vi "Read_Config.vi"(0 "GPIO 1 Config":enum32{"Off", "Read", "Write", "PWM "}(radio), 1 "GPIO 2 Config":enum32{"Off", "Read", "Write", "PWM "}(radio), 2 "GPIO 3 Config":enum32{"Off", "Read", "Write", "PWM "}(radio), 3 "Battery_Config":u16(ring)=1 items=["Off", "On"], 6 "Analog 1 Config":enum32{"Analog Read", "Off"}(radio), 10 "Analog 2 Config":enum32{"Analog Read", "Off"}(radio), 11 "Analog 3 Config":enum32{"Analog Read", "Off"}(radio), 14 "Error In":errorcluster, 15 "LINX Resource":T1) -> (18 "Read_Config":i32[](array[numeric]), 19 "Voltage":dbl(slide) caption="Tank" scale=3.0..6.0, 20 "GPIO 1 Read":bool, 21 "Analog 2":dbl, 22 "GPIO 2 Read":bool, 23 "Analog 3":dbl, 24 "GPIO 3 Read":bool, 25 "Error Out":errorcluster, 26 "Analog 1":dbl, 27 "LINX Resource 2":T1)   [LabVIEW 2018, in "ArgoBotLib.lvlib"]
uses:
  ArgoBotLib.lvlib
  <vilib>/MakerHub/LINX/Private/Type Defs/LINX Ref.ctl
  <vilib>/MakerHub/LINX/Private/Type Defs/Platform.ctl
  <vilib>/MakerHub/LINX/Private/Type Defs/Interface.ctl
  <vilib>/MakerHub/LINX/Private/Device/Type Defs/LINX Device Config.ctl
  <vilib>/MakerHub/LINX/Private/Device/Type Defs/TCP Config.ctl
  <vilib>/MakerHub/LINX/Private/Device/Type Defs/Channels.ctl
  <vilib>/MakerHub/LINX/Public/Peripherals/Digital/Digital Read N Chans.vi
  <vilib>/MakerHub/LINX/Public/Peripherals/Analog/Analog Read N Chans.vi
  <vilib>/MakerHub/LINX/Private/Local IO/LinxDigitalRead.vi
  <vilib>/MakerHub/LINX/Public/Utilities/Check Channel.vi
  <vilib>/MakerHub/LINX/Private/Local IO/LinxAnalogRead.vi
  <vilib>/MakerHub/LINX/Private/Utilties/Generate Error.vi
  <vilib>/MakerHub/LINX/LMH-LINX.lvlib
  <vilib>/MakerHub/LINX/Private/Device/Device.lvlib
panel:
  # "ArgoBot Read Config"
  # "This vi configures and reads the gpio and analog channels"
  # "Inputs"
  # "Outputs"
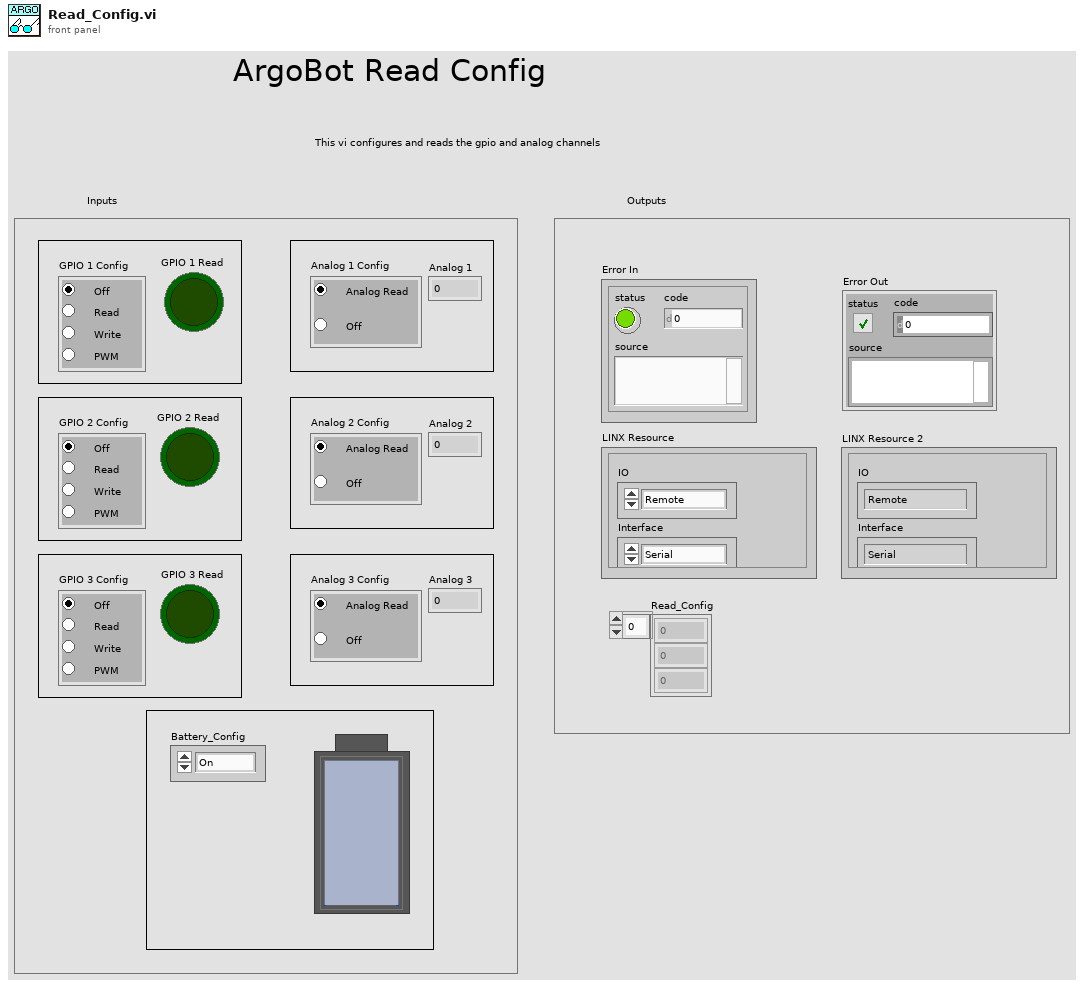
[diagram p1: front panel]
types:
  T1 = typedef "LMH-LINX.lvlib/LINX Ref.ctl" = cluster{"IO":T2, "Interface":T3, "LINX Device Config":T4}
  T2 = typedef "LMH-LINX.lvlib/Platform.ctl" = enum16{"Remote", "Local"}
  T3 = typedef "LMH-LINX.lvlib/Interface.ctl" = enum16{"Serial", "TCP"}
  T4 = typedef "LMH-LINX.lvlib/Device.lvlib/LINX Device Config.ctl" = cluster{"Interface":T3, "COM Port":refnum<visa-resource-name>, "TCP Configuration":T5, "Device Family":u8, "Device ID":u8, "Device Name":string, "TCP Ref":refnum<k5>, "Channels":T6}
  T5 = typedef "LMH-LINX.lvlib/Device.lvlib/TCP Config.ctl" = cluster{"IP Address":string, "Port":u16}
  T6 = typedef "LMH-LINX.lvlib/Channels.ctl" = cluster{"DI":u8[], "DO":u8[], "AI":u8[], "AO":u8[], "PWM":u8[], "QE":u8[], "UART":u8[], "I2C 2":u8[], "SPI":u8[], "CAN":u8[], "Servo":u8[], "AI Ref (V)":dbl, "AI Resolution (Bits)":u8, "AO Ref (V)":dbl, "AO Resolution (Bits)":u8}
  T7 = cluster{"GPIO 1 Config":enum32{"Off", "Read", "Write", "PWM "}, "GPIO 2 Config":enum32{"Off", "Read", "Write", "PWM "}, "GPIO 3 Config":enum32{"Off", "Read", "Write", "PWM "}, "Analog 1 Config":enum32{"Analog Read", "Off"}, "Analog 2 Config":enum32{"Analog Read", "Off"}, "Analog 3 Config":enum32{"Analog Read", "Off"}, "Battery_Config":u16, "LINX Resource":T1, "Error In":errorcluster}
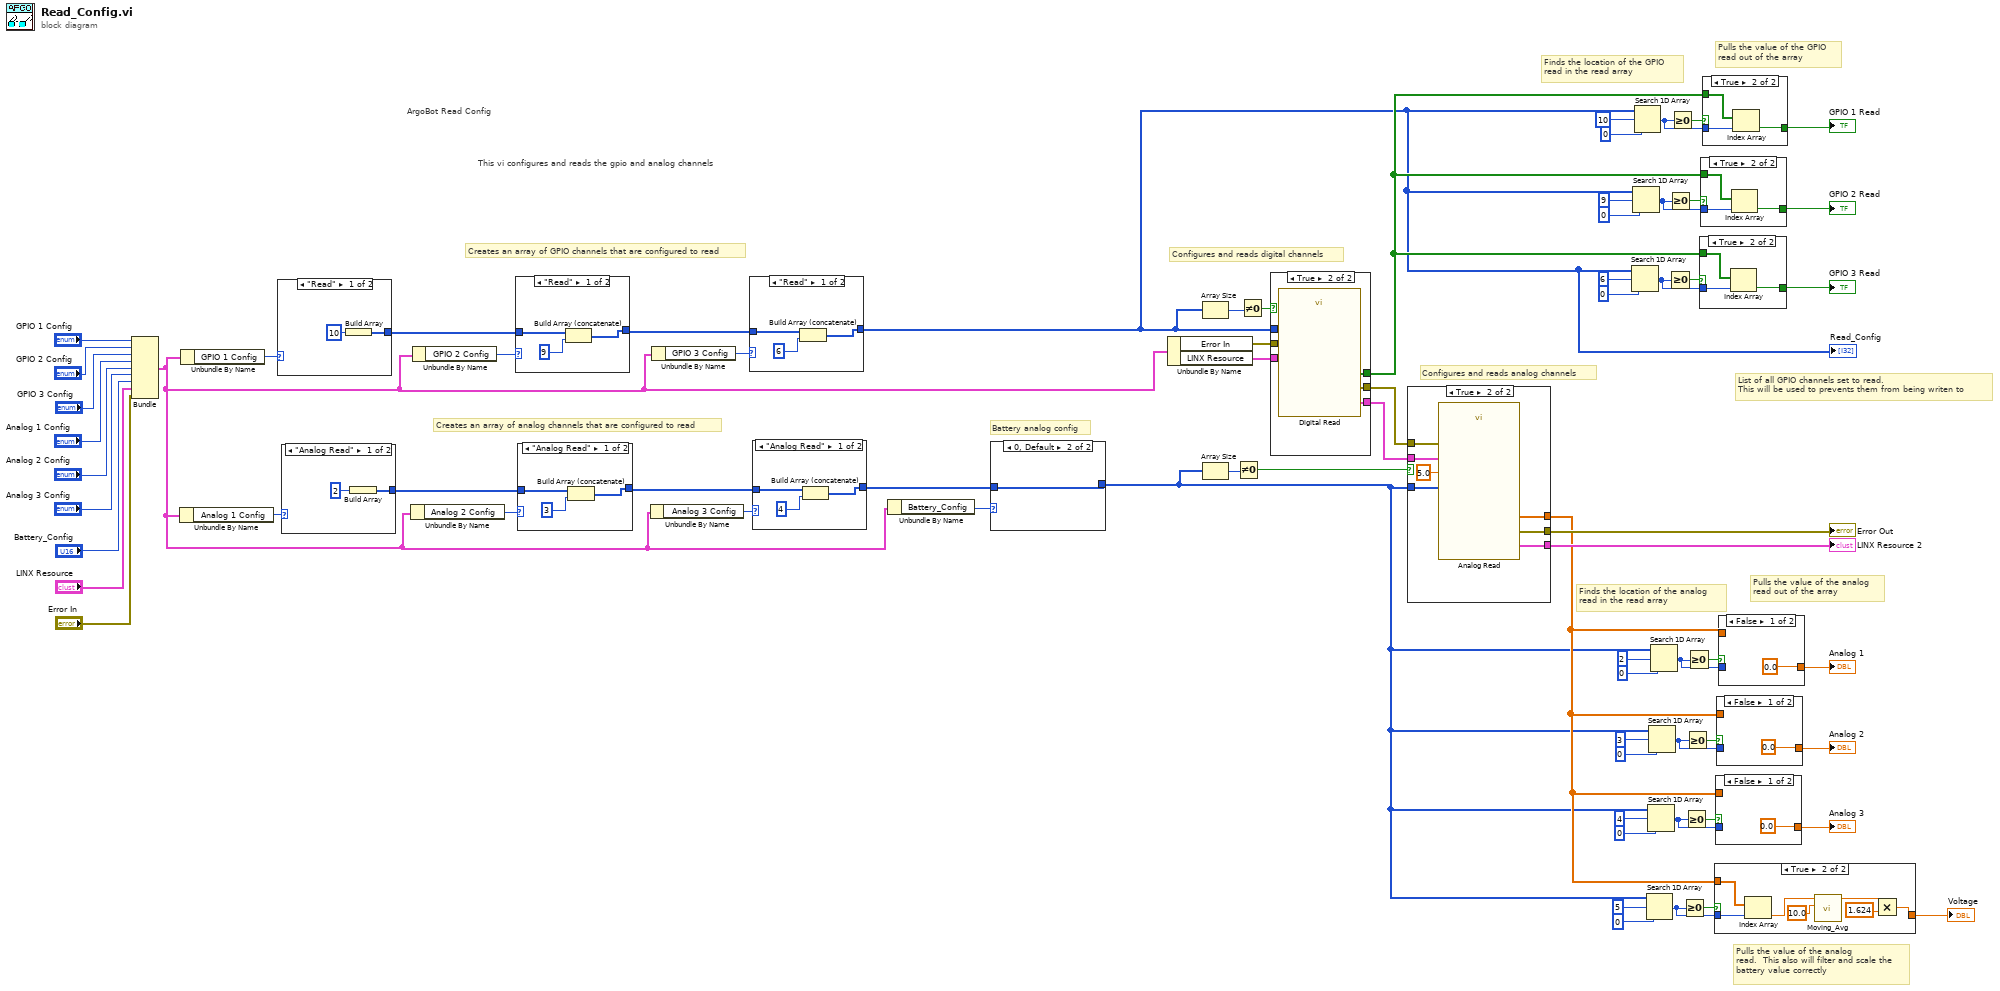
[diagram p0: block diagram]
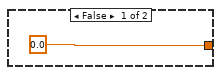
[diagram p2: hidden frame]
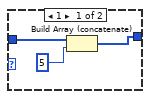
[diagram p3: hidden frame]
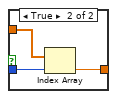
[diagram p4: hidden frame]
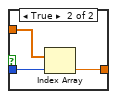
[diagram p5: hidden frame]
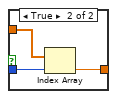
[diagram p6: hidden frame]
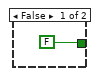
[diagram p7: hidden frame]
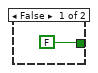
[diagram p8: hidden frame]
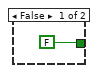
[diagram p9: hidden frame]
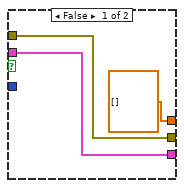
[diagram p10: hidden frame]
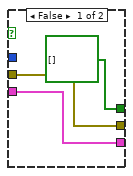
[diagram p11: hidden frame]
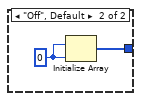
[diagram p14: hidden frame]
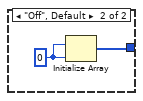
[diagram p17: hidden frame]
diagram:
  # "List of all GPIO channels set to read.  \nThis will be used to prevents them from being writen to"
  # "Pulls the value of the analog \nread.  This also will filter and scale the \nbattery value correctly"
  # "Pulls the value of the analog \nread out of the array"
  # "Pulls the value of the GPIO \nread out of the array"
  # "Finds the location of the analog \nread in the read array"
  # "Finds the location of the GPIO \nread in the read array"
  # "Configures and reads analog channels"
  # "Configures and reads digital channels"
  # "Battery analog config"
  # "Creates an array of analog channels that are configured to read"
  # "Creates an array of GPIO channels that are configured to read"
  # "This vi configures and reads the gpio and analog channels"
  # "ArgoBot Read Config"
  n1 = Bundle("GPIO 1 Config"="GPIO 1 Config", "GPIO 2 Config"="GPIO 2 Config", "GPIO 3 Config"="GPIO 3 Config", "Analog 1 Config"="Analog 1 Config", "Analog 2 Config"="Analog 2 Config", "Analog 3 Config"="Analog 3 Config", "Battery_Config"="Battery_Config", "LINX Resource"="LINX Resource", "Error In"="Error In") -> (w4:T7)  [unwired: 1 in]
  n2 = Unbundle By Name(w4) -> ("Analog 1 Config"=w59:enum32{"Analog Read", "Off"})
  n3 = Unbundle By Name(w4) -> ("GPIO 1 Config"=w68:enum32{"Off", "Read", "Write", "PWM "})
  n4 = case shown="\"Read\"" w68 {
    tunnel: [w73 w75] -> w66
    frame "Read" {
      n5 = Build Array(10) -> (w73:i32[])
    }
    frame "Off", Default {
      w74 = 0 ("dimension size")
      n6 = Initialize Array(w74, w74) -> (w75:i32[])
    }
  }
  n7 = case shown="\"Analog Read\"" w59 {
    tunnel: [w77 w78] -> w62
    frame "Analog Read" {
      n8 = Build Array(2) -> (w77:i32[])
    }
    frame "Off", Default {
      w79 = 0 ("dimension size")
      n9 = Initialize Array(w79, w79) -> (w78:i32[])
    }
  }
  n10 = Unbundle By Name(w4) -> ("Analog 2 Config"=w63:enum32{"Analog Read", "Off"})
  n11 = Unbundle By Name(w4) -> ("GPIO 2 Config"=w67:enum32{"Off", "Read", "Write", "PWM "})
  n12 = case shown="\"Read\"" w67 {
    tunnel: [w81 w83] -> w64
    tunnel: w66 -> [w82 w83]
    frame "Read" {
      n13 = Build Array (concatenate)(w82, 9) -> (w81:i32[])
    }
    frame "Off", Default {
    }
  }
  n14 = case shown="\"Analog Read\"" w63 {
    tunnel: [w85 w87] -> w60
    tunnel: w62 -> [w86 w87]
    frame "Analog Read" {
      n15 = Build Array (concatenate)(w86, 3) -> (w85:i32[])
    }
    frame "Off", Default {
    }
  }
  n16 = Unbundle By Name(w4) -> ("Analog 3 Config"=w61:enum32{"Analog Read", "Off"})
  n17 = Unbundle By Name(w4) -> ("GPIO 3 Config"=w65:enum32{"Off", "Read", "Write", "PWM "})
  n18 = case shown="\"Read\"" w65 {
    tunnel: [w89 w91] -> w14
    tunnel: w64 -> [w90 w91]
    frame "Read" {
      n19 = Build Array (concatenate)(w90, 6) -> (w89:i32[])
    }
    frame "Off", Default {
    }
  }
  "Read_Config" <- w14
  n20 = case shown="\"Analog Read\"" w61 {
    tunnel: [w93 w95] -> w13
    tunnel: w60 -> [w94 w95]
    frame "Analog Read" {
      n21 = Build Array (concatenate)(w94, 4) -> (w93:i32[])
    }
    frame "Off", Default {
    }
  }
  n22 = Unbundle By Name(w4) -> ("Battery_Config"=w3:u16)
  n23 = case shown="0, Default" w3 {
    tunnel: [w97 w99] -> w7
    tunnel: w13 -> [w98 w99]
    frame 1 {
      n24 = Build Array (concatenate)(w98, 5) -> (w97:i32[])
    }
    frame 0, Default {
    }
  }
  n25 = Unbundle By Name(w4) -> ("Error In"=w56:errorcluster, "LINX Resource"=w55:T1)
  n26 = Array Size(array=w14) -> (size(s)=w23:i32)
  n27 = Array Size(array=w7) -> (size(s)=w21:i32)
  n28 = Not Equal To 0?(x=w21) -> (x != 0?=w54:bool)
  n29 = Not Equal To 0?(x=w23) -> (x != 0?=w22:bool)
  n30 = case shown="True" w22 {
    tunnel: w14 -> [_ w108]
    tunnel: [w102 w107] -> w58
    tunnel: [w101 w106] -> w57
    tunnel: w56 -> [w102 w105]
    tunnel: w55 -> [w101 w104]
    tunnel: [bool[] [] ("Values") w103] -> w20
    frame False {
    }
    frame True {
      n31 = call-poly <vilib>:"Digital Read.vi"("Error In"=w105, "DI Channels"=w108, "LINX Resource"=w104) -> ("Error Out"=w107:errorcluster, "Values"=w103:bool[], "LINX Resource"=w106:T1)  [unwired: 6 in]
    }
  }
  n32 = case shown="True" w54 {
    tunnel: w58 -> [w111 w118]
    tunnel: w57 -> [w110 w117]
    tunnel: w7 -> [_ w115]
    tunnel: [w111 w114] -> w53
    tunnel: [w110 w113] -> w52
    tunnel: [dbl[] [] ("Voltages") w112] -> w8
    frame False {
    }
    frame True {
      n33 = call-poly <vilib>:"Analog Read.vi"("Analog Ref Override"=5.0, "Error In"=w118, "AI Channel(s)"=w115, "LINX Resource"=w117) -> ("Error Out"=w114:errorcluster, "Voltages"=w112:dbl[], "LINX Resource"=w113:T1)  [unwired: 4 in, 1 out]
    }
  }
  "Error Out" <- w53
  "LINX Resource 2" <- w52
  n34 = Search 1D Array(1D array=w14, element=6, start index (0)=0) -> (index of element=w42:i32)
  n35 = Search 1D Array(1D array=w14, element=9, start index (0)=0) -> (index of element=w43:i32)
  n36 = Search 1D Array(1D array=w14, element=10, start index (0)=0) -> (index of element=w48:i32)
  n37 = Search 1D Array(1D array=w7, element=5, start index (0)=0) -> (index of element=w12:i32)
  n38 = Search 1D Array(1D array=w7, element=4, start index (0)=0) -> (index of element=w35:i32)
  n39 = Search 1D Array(1D array=w7, element=3, start index (0)=0) -> (index of element=w34:i32)
  n40 = Search 1D Array(1D array=w7, element=2, start index (0)=0) -> (index of element=w30:i32)
  n41 = Greater Or Equal To 0?(x=w42) -> (x >= 0?=w41:bool)
  n42 = Greater Or Equal To 0?(x=w43) -> (x >= 0?=w44:bool)
  n43 = Greater Or Equal To 0?(x=w48) -> (x >= 0?=w49:bool)
  n44 = Greater Or Equal To 0?(x=w12) -> (x >= 0?=w11:bool)
  n45 = Greater Or Equal To 0?(x=w35) -> (x >= 0?=w36:bool)
  n46 = Greater Or Equal To 0?(x=w34) -> (x >= 0?=w33:bool)
  n47 = Greater Or Equal To 0?(x=w30) -> (x >= 0?=w29:bool)
  n48 = case shown="True" w41 {
    tunnel: w42 -> [_ w122]
    tunnel: w20 -> [_ w121]
    tunnel: [FALSE w120] -> w18
    frame False {
    }
    frame True {
      n49 = Index Array(array=w121, index=w122) -> (element=w120:bool)
    }
  }
  "GPIO 3 Read" <- w18
  n50 = case shown="True" w44 {
    tunnel: w43 -> [_ w126]
    tunnel: w20 -> [_ w125]
    tunnel: [FALSE w124] -> w19
    frame False {
    }
    frame True {
      n51 = Index Array(array=w125, index=w126) -> (element=w124:bool)
    }
  }
  "GPIO 2 Read" <- w19
  n52 = case shown="True" w49 {
    tunnel: w48 -> [_ w130]
    tunnel: w20 -> [_ w129]
    tunnel: [FALSE w128] -> w47
    frame False {
    }
    frame True {
      n53 = Index Array(array=w129, index=w130) -> (element=w128:bool)
    }
  }
  "GPIO 1 Read" <- w47
  n54 = case shown="True" w11 {
    tunnel: w12 -> [_ w138]
    tunnel: w8 -> [_ w137]
    tunnel: [0.0 w133] -> w1
    frame False {
    }
    frame True {
      n55 = Index Array(array=w137, index=w138) -> (element=w136:dbl)
      n56 = call "Moving_Avg.vi"("Num_Avg"=10.0, "Numeric in"=w136) -> ("Numeric out"=w134:dbl)  [unwired: 9 in]
      n57 = Multiply(x=w134, y=1.624 ("Num_Avg")) -> (x*y=w133:dbl)
    }
  }
  "Voltage" <- w1
  n58 = case shown="False" w36 {
    tunnel: w35 -> [_ w142]
    tunnel: w8 -> [_ w141]
    tunnel: [0.0 w140] -> w24
    frame False {
    }
    frame True {
      n59 = Index Array(array=w141, index=w142) -> (element=w140:dbl)
    }
  }
  "Analog 3" <- w24
  n60 = case shown="False" w33 {
    tunnel: w34 -> [_ w146]
    tunnel: w8 -> [_ w145]
    tunnel: [0.0 w144] -> w25
    frame False {
    }
    frame True {
      n61 = Index Array(array=w145, index=w146) -> (element=w144:dbl)
    }
  }
  "Analog 2" <- w25
  n62 = case shown="False" w29 {
    tunnel: w30 -> [_ w150]
    tunnel: w8 -> [_ w149]
    tunnel: [0.0 w148] -> w26
    frame False {
    }
    frame True {
      n63 = Index Array(array=w149, index=w150) -> (element=w148:dbl)
    }
  }
  "Analog 1" <- w26
